vi "Test_BufferedLogAddSink_NoErrorReturned.vi"(8 "error in (no error)":errorcluster, 11 "TestCase in":refnum<class "TestBufferedLogSink.lvclass">) -> (0 "error out":errorcluster, 3 "TestCase out":refnum<class "TestBufferedLogSink.lvclass">)   [LabVIEW 2019, in "TestBufferedLogSink.lvclass"]
uses:
  TestBufferedLogSink.lvclass
  Source/Composed Log/LoggerReference/LoggerReference.lvclass/LoggerReference.ctl
  b83ac39a-525a-4956-83d8-1e446c51aff0.vi
  Source/Composed Log/LoggerReference/Return Aggregate Queues.vi
  Source/Composed Log/LoggerReference/Add Aggregate Log.vi
  b83ac39a-525a-4956-83d8-1e446c51aff0.vi/f4672d8b-dd16-4b18-9c5d-995299dd5836.vi
  Source/Composed Log/LoggerReference/Send Add Sink.vi
  Source/LVQueue Sink/LVQueue Sink.lvclass
  C:/CS/Log/Source/Composed Log/Log Sink/Log Sink.lvclass
  Source/Buffered Log Sink/Buffered Log Sink.lvclass
  Source/Composed Log/Application Logger/Launch Worker Loop.vi
  Source/Composed Log/LoggerReference/Initialize Logger Instance.vi
  Source/Composed Log/LoggerReference/LoggerReference.lvclass
  Source/Composed Log/IErrorFormat/IErrorFormat.lvclass
  Source/Composed Log/Log Sink/Log Sink.lvclass
  <vilib>/addons/_JKI Toolkits/VI Tester/TestCase.llb/TestCase.lvclass
  C:/Program Files (x86)/National Instruments/LabVIEW 2019/vi.lib/addons/_JKI Toolkits/VI Tester/TestCase.llb/TestCase.lvclass
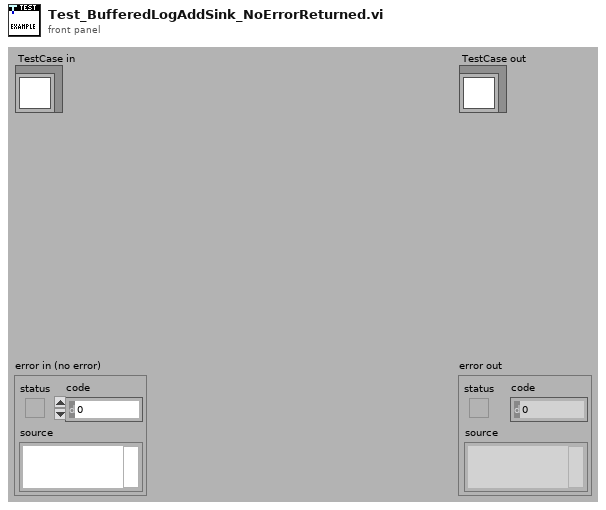
[diagram p1: front panel]
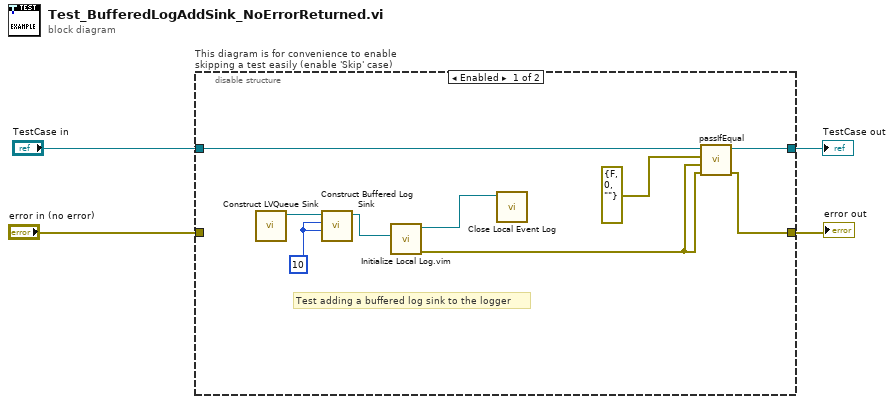
[diagram p0: block diagram]
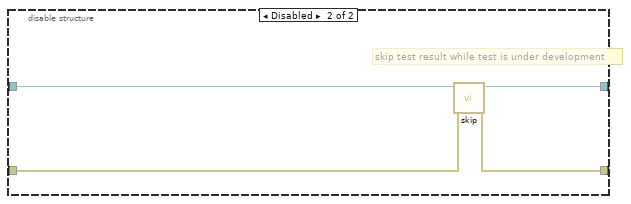
[diagram p2: hidden frame]
diagram:
  n1 = disable-structure "This diagram is for convenience to enable skipping a test easily (enable 'Skip' case)" shown="Enabled" {
    disable-tunnel: "TestCase in" -> [w10 w17]
    disable-tunnel: [w6 w15] -> w1
    disable-tunnel: [w9 w16] -> w3
    disable-tunnel: "error in (no error)" -> [_ w14]
    frame Enabled {
      w11 = 10 ("Buffer Timeout ms (-1)")
      # "Test adding a buffered log sink to the logger"
      n2 = call "Construct LVQueue Sink.vi"() -> ("LVQueue Sink out"=w12:refnum<class "LVQueue Sink.lvclass">)  [unwired: 10 in, 1 out]
      n3 = call "Construct Buffered Log Sink.vi"("Buffer Size (128)"=w11, "Buffer Timeout ms (-1)"=w11, "Sink to Buffer"=w12) -> ("Buffered Log Sink out"=w5:refnum<class "Buffered Log Sink.lvclass">)  [unwired: 8 in]
      n4 = call "Initialize Local Log.vim"("Startup Sink(s)"=w5) -> ("error out"=w8:errorcluster, "Log Instance Reference"=w13:refnum<class "LoggerReference.lvclass">)  [unwired: 8 in, 1 out]
      n5 = call "Close Local Event Log.vi"("Log Instance"=w13) -> ()  [unwired: 10 in, 1 out]
      n6 = call-dynamic "passIfEqual.vi"("error in (no error)"=w8, "y"=w8, "x"=errorcluster {"status"=FALSE, "code"=0, "source"=""} ("error out"), "TestCase in"=w10) -> ("error out"=w9:errorcluster, "TestCase out"=w6:refnum<class "TestBufferedLogSink.lvclass">)  [unwired: 6 in]
    }
    frame Disabled {
      # "skip test result while test is under development"
      n7 = call <vilib>:"skip.vi"("error in (no error)"=w14, "TestCase in"=w17) -> ("error out"=w16:errorcluster, "TestCase out"=w15:refnum<class "TestBufferedLogSink.lvclass">)  [unwired: 8 in]
    }
  }
  "error out" <- w3
  "TestCase out" <- w1
